vi "Run.vi"(8 "Error In":errorcluster) -> (0 "Error Out":errorcluster)   [LabVIEW 2014, in "Logger.lvlib"]
uses:
  Logger.lvlib
  Private/File/_Action.ctl
  Private/_Control Action.ctl
  Private/File/File.lvlib
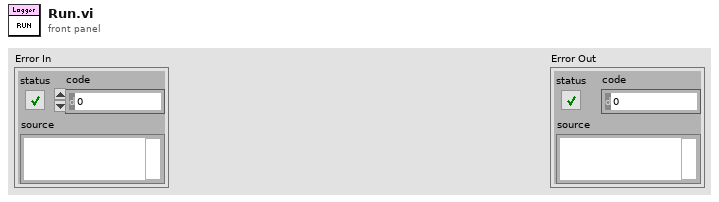
[diagram p1: front panel]
types:
  T1 = typedef "Logger.lvlib/File.lvlib/_Action.ctl" = enum16{"Initialize", "Set File Size Limit", "Set Root Folder", "Start", "Write", "Stop", "Shutdown"}
  T2 = typedef "Logger.lvlib/_Control Action.ctl" = enum16{"Initialize", "Get", "Set", "Shutdown"}
  T3 = typedef "LV-Logger.lvlib/Message.ctl" = cluster{"Time Stamp":timestamp, "Tag":T4, "Source":string, "Text":string}
  T4 = typedef "LV-Logger.lvlib/Tag.ctl" = enum16{"Fatal", "Error", "Warn", "Info", "Debug", "Trace"}
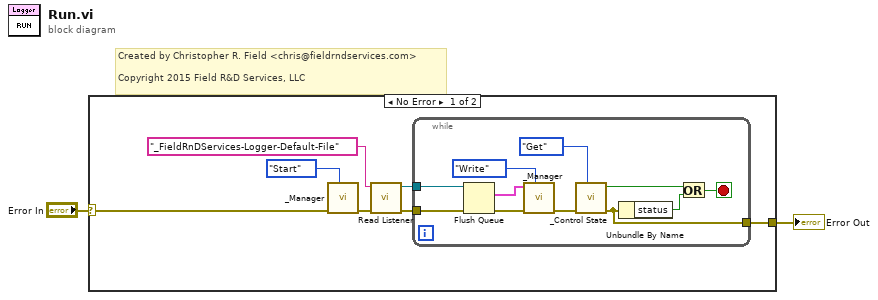
[diagram p0: block diagram]
diagram:
  # "Created by Christopher R. Field <chris@fieldrndservices.com>\n\nCopyright 2015 Field R&D Services, LLC"
  n1 = case shown="No Error" "Error In" {
    selector: "Error In" -> [w8 w21]
    tunnel: [w4 w21] -> w1
    frame No Error {
      n2 = call "_Manager.vi"("Action"=_Action."Start", "Error In"=w8) -> ("Error Out"=w7:errorcluster)  [unwired: 9 in]
      n3 = call "Read Listener.vi"("Error In"=w7, "Listener ID"="_FieldRnDServices-Logger-Default-File") -> ("Error Out"=w5:errorcluster, "Listener"=w6:refnum<queue>)  [unwired: 8 in]
      n4 = while {
        tunnel: w6 -> [w20]
        tunnel: w5 -> [w19]
        tunnel: [w14] -> w4
        stop <- w10 stop-if-true
        n5 = Flush Queue(queue=w20, error in (no error)=w19) -> (remaining elements=w18:T3[], error out=w17:errorcluster)  [unwired: 1 out]
        n6 = call "_Manager.vi"("Action"=_Action."Write", "Error In"=w17, "Set Value"=w18) -> ("Error Out"=w15:errorcluster)  [unwired: 8 in]
        n7 = call "_Control State.vi"("Action"=_Control_Action."Get", "Error In"=w15) -> ("Error Out"=w14:errorcluster, "Stop?"=w11:bool)  [unwired: 8 in]
        n8 = Unbundle By Name(w14) -> ("status"=w12:bool)
        n9 = Or(x=w11, y=w12) -> (x .or. y?=w10:bool)
      }
    }
    frame Error {
    }
  }
  "Error Out" <- w1
